vi "runHTTemperature.vi"() -> ()   [LabVIEW 2012]
uses:
  <vilib>/Utility/file.llb/Read From Spreadsheet File (string).vi
  <vilib>/regexp/Match Regular Expression.xnode
panel:
  out "error out":errorcluster
  out "concatenated string 2":string
  in  "file path (dialog if empty)":path=path "C:/temp/ht/now/HTentity.txt"
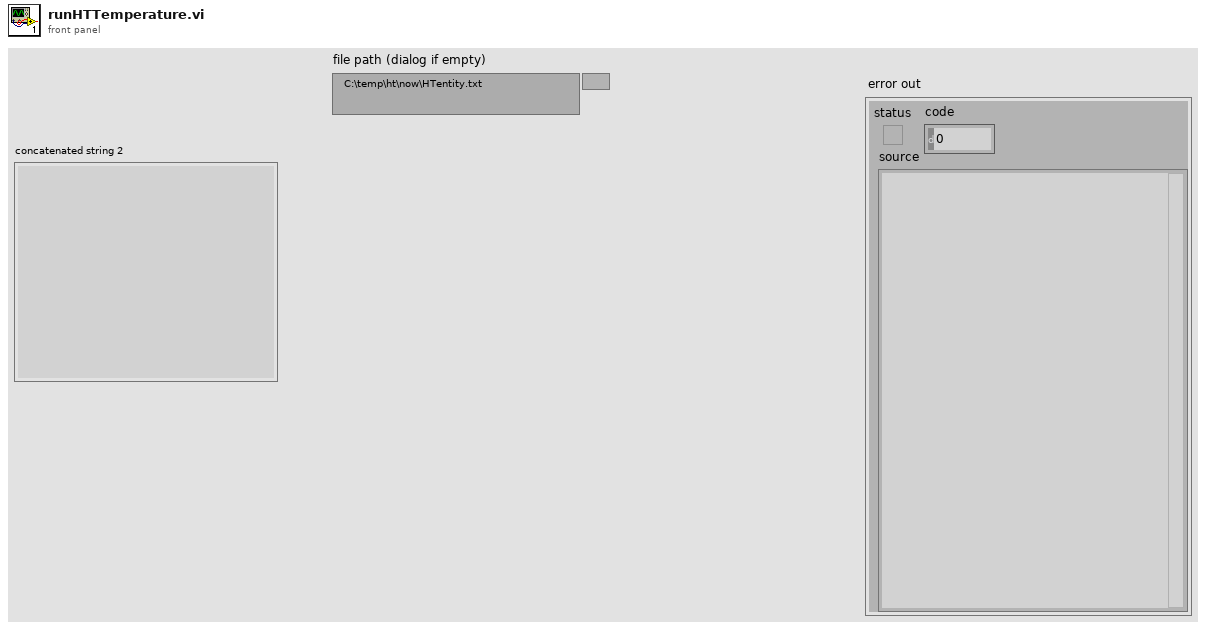
[diagram p1: front panel]
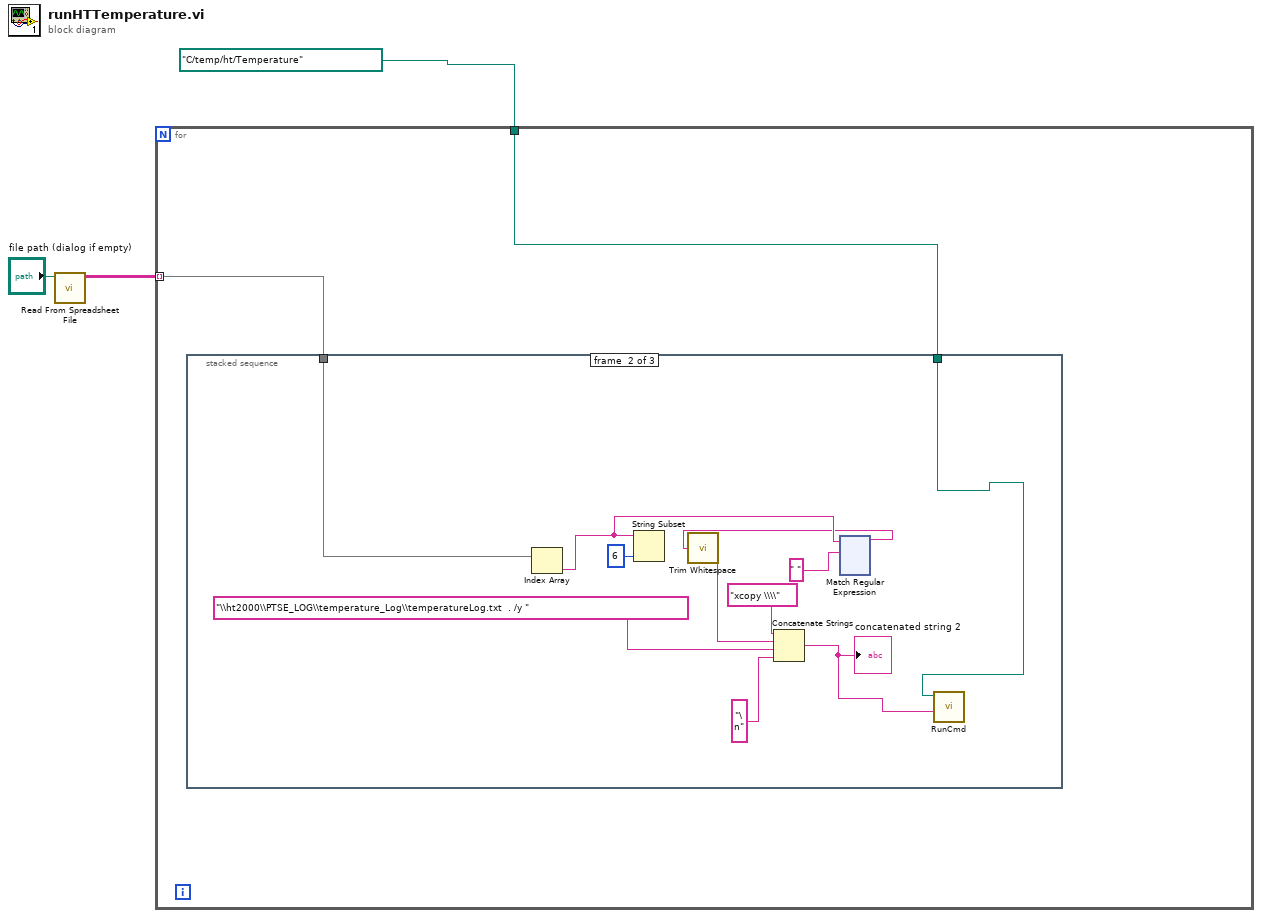
[diagram p0: block diagram]
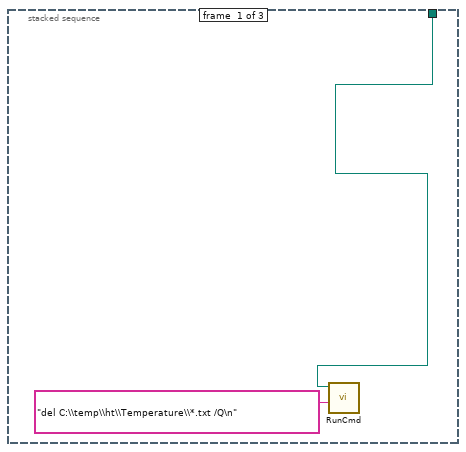
[diagram p2: hidden frame]
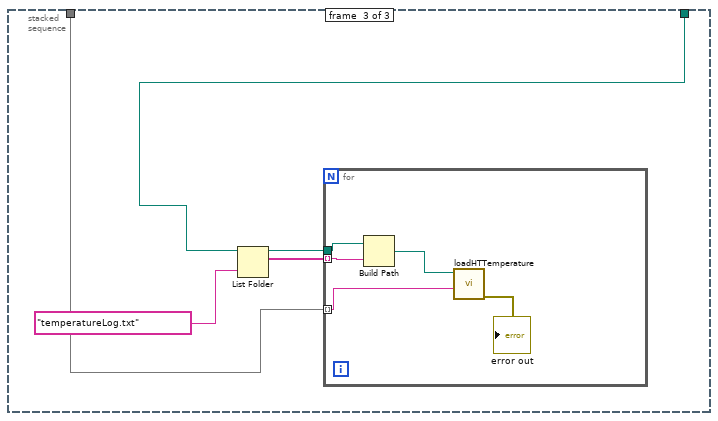
[diagram p3: hidden frame]
diagram:
  n1 = call-poly <vilib>:"Read From Spreadsheet File.vi"("file path (dialog if empty)"="file path (dialog if empty)") -> ("all rows"=w2:string[][])  [unwired: 6 in, 4 out]
  n2 = for {
    tunnel: w2 -> [w5] mode=indexing
    tunnel: path "C:/temp/ht/Temperature" ("path") -> [w4]
    n3 = stacked-sequence {
      tunnel: w5 -> [_ w10 w130]
      tunnel: w4 -> [w6 w9 w131]
      frame #0 {
        n4 = call "RunCmd.vi"("Cmd String"="del C:\\temp\\ht\\Temperature\\*.txt /Q\n", "working directory"=w6) -> ()  [unwired: 8 in, 2 out]
      }
      frame #1 {
        n5 = Index Array(array=w10) -> (element=w14:string)  [unwired: 1 in]
        n6 = String Subset(string=w14, length (rest)=6 ("length (rest)")) -> ()  [unwired: 1 in, 1 out]
        n7 = xnode "Match Regular Expression"("input string"=w14, "regular expression"=" ") -> ("before match"=w13:string)  [unwired: 4 in, 4 out]
        n8 = call <vilib>:"Trim Whitespace.vi"("string"=w13) -> ("trimmed string"=w11:string)  [unwired: 1 in]
        n9 = Concatenate Strings("xcopy \\\\" ("string"), w11, "\\ht2000\\PTSE_LOG\\temperature_Log\\temperatureLog.txt  . /y " ("string"), "\n" ("string")) -> (w17:string)
        "concatenated string 2" <- w17
        n10 = call "RunCmd.vi"("Cmd String"=w17, "working directory"=w9) -> ()  [unwired: 8 in, 2 out]
      }
      frame #2 {
        n11 = List Folder(path=w131, pattern="temperatureLog.txt") -> (path out=w133:path, filenames=w132:string[])  [unwired: 2 in, 2 out]
        n12 = for {
          tunnel: w133 -> [w139]
          tunnel: w132 -> [w138] mode=indexing
          tunnel: w130 -> [w136] mode=indexing
          n13 = Build Path(base path=w139, name or relative path=w138) -> (appended path=w137:path)
          n14 = call "loadHTTemperature.vi"("Entity"=w136, "file (use dialog)"=w137) -> ("error out"=→"error out":errorcluster)  [unwired: 9 in]
        }
      }
    }
  }
